vi "GetFrameFFT_index.vi"(7 "sframe Max":i32=2, 11 "element":T1) -> (1 "average series":i32, 3 "index out":i32)   [LabVIEW 2018]
uses:
  typedef/AcquisitionFrame.ctl
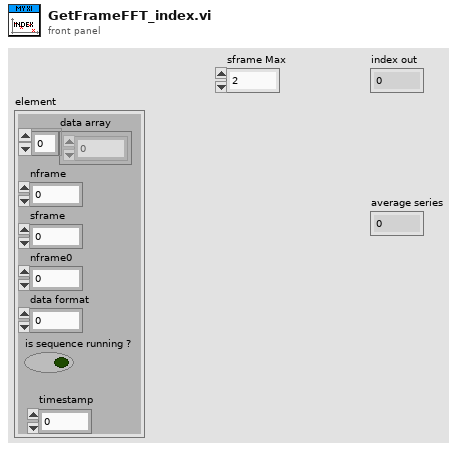
[diagram p1: front panel]
types:
  T1 = typedef "AcquisitionFrame.ctl" = cluster{"data array":u8[], "nframe":i32, "sframe":i32, "nframe0":i32, "data format":i32, "is sequence running ?":bool, "timestamp":dbl}
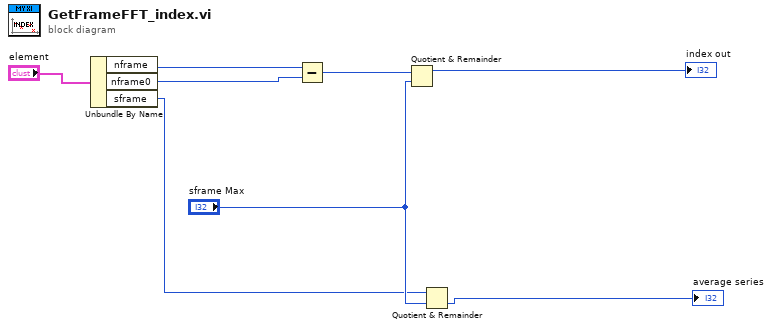
[diagram p0: block diagram]
diagram:
  n1 = Unbundle By Name("element") -> ("nframe"=w3:i32, "nframe0"=w2:i32, "sframe"=w1:i32)
  n2 = Subtract(x=w3, y=w2) -> (x-y=w8:i32)
  n3 = Quotient & Remainder(x=w8, y="sframe Max") -> (x-y*floor(x/y)=→"index out":i32)  [unwired: 1 out]
  n4 = Quotient & Remainder(x=w1, y="sframe Max") -> (floor(x/y)=→"average series":i32)  [unwired: 1 out]
